vi "Write Y.vi"(2 "error in (no error)":errorcluster, 3 "Y":dbl, 4 "Sensor In":refnum<class "Sensor.lvclass">) -> (0 "error out":errorcluster, 1 "Sensor Out":refnum<class "Sensor.lvclass">)   [LabVIEW 2015, in "Sensor.lvclass"]
uses:
  Sensor.lvclass
  Sensor.lvclass/Sensor.ctl
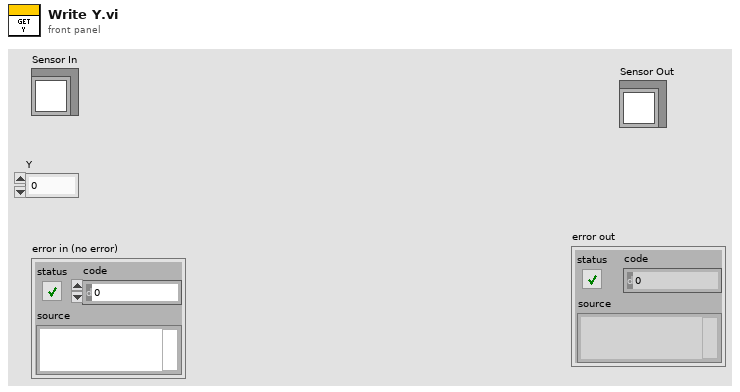
[diagram p1: front panel]
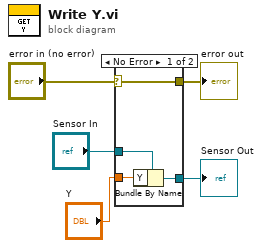
[diagram p0: block diagram]
diagram:
  n1 = case shown="No Error" "error in (no error)" {
    selector: "error in (no error)" -> [w9 w10]
    tunnel: [w9 w10] -> w4
    tunnel: "Sensor In" -> [w8 w11]
    tunnel: "Y" -> [w7 _]
    tunnel: [w6 w11] -> w1
    frame No Error {
      n2 = Bundle By Name(cluster=w8, "Y"=w7) -> (w6:refnum<class "Sensor.lvclass">)
    }
    frame Error {
    }
  }
  "Sensor Out" <- w1
  "error out" <- w4
